vi "_SendTelemetry.vi"(5 "Bytes":u8, 6 "Output":refnum<k21>, 7 "Telemetry Offset":i16, 8 "error in (no error)":errorcluster, 9 "IP in":i16, 10 "Instructions":refnum<k21>, 11 "Telemetry FIFO":refnum<k21>) -> (0 "error out":errorcluster, 3 "IP out":i16)   [LabVIEW 2018, in "Modbus_Processing_Unit.lvlib" / "MPU.lvclass"]
uses:
  MPU.lvclass
  ts_m1m3supportFPGA/src/Common_FPGA_HealthAndStatus/DataTypes/HealthAndStatusUpdate.ctl
  ts_m1m3supportFPGA/src/Common_FPGA_HealthAndStatus/DataTypes/HealthAndStatusUpdateMode.ctl
  <vilib>/rvi/DataTransferAndStorage/Container/Common/niFpgaContainerExecOnDevCompGetState.vi
  <vilib>/rvi/Emulation/niFpgaEmulationIsFPGAContextNoSignature.vi
  <vilib>/rvi/DataTransferAndStorage/Container/Common/niFpgaContainerGetUniqueNameForEmu.vi
  <vilib>/rvi/Emulation/niFpgaProcessEmulError.vi
  <vilib>/rvi/Emulation/niFpgaSctlEmulationGetInTimedLoop.vi
  <vilib>/rvi/errors/nirviReportUnexpectedCaseInternalError (U32).vi
  <vilib>/rvi/Memory/Memory_Emulation/niFpgaMemoryEmulationCacheClearOnFirstRun.vi
  <vilib>/rvi/Memory/Memory_Emulation/nirvimemoryEmulationManagerCache_MakeExclusive.vi
  <vilib>/rvi/Memory/Memory_Emulation/niFpgaMemoryEmulationValidateCache.vi
  <vilib>/rvi/Memory/Memory_Emulation/nirvimemoryEmulationManagerCache_InsertValue.vi
  <vilib>/Utility/error.llb/Clear Errors.vi
  <vilib>/rvi/Memory/Memory_Emulation/nirvimemoryEmulationManagerCache_ReleaseExclusive.vi
  <vilib>/rvi/Memory/Memory_Emulation/nirvimemoryEmulationManagerCache_GetValue.vi
  <vilib>/rvi/Memory/Memory_Emulation/nirvimemoryEmulationManagerCache_SetValue.vi
  <vilib>/rvi/Emulation/niFpgaSctlEmulationResourceMgr.vi
  <vilib>/rvi/errors/niFpgaSetErrorForExecOnDevCompSimple.vi
  <vilib>/rvi/eio/common/nirviEmuReportErrorAndStop.vi
  <vilib>/rvi/FIFO/Fifo_Resource/nirvififoEmulationSetSize.vi
  <vilib>/rvi/FIFO/Fifo_Resource/nirviFifoEmulationQueueMgr.vi
  <instcachedir>/0/nirviFifoEmulationQueueMgr_E5CAEC123FF24DC58D834DCA3CDAA9B5.lvgen/nirviFifoEmulationQueueMgr_E5CAEC123FF24DC58D834DCA3CDAA9B5_022.vi
  <vilib>/rvi/FIFO/Fifo_Resource/nirvififoEmulationDetermineInputValidOut.vi
  <vilib>/rvi/FIFO/Fifo_Resource/nirvififoEmulationCreateLock.vi
  <vilib>/rvi/FIFO/Fifo_Resource/nirvififoEmulationObtainLock.vi
  <vilib>/rvi/FIFO/Fifo_Resource/nirvififoEmulationReleaseLock.vi
  <vilib>/rvi/occurrence/nirviWaitOnOccurrenceBase.vi
  <vilib>/rvi/errors/nirviReportUnexpectedCaseInternalError.vi
  <vilib>/rvi/interface/RandomDataEmulation/niFpgaRandomDataHandleErrors.vi
  <vilib>/rvi/DataTransferAndStorage/Container/XNode/niFpgaContainer.xnode
  <vilib>/rvi/Memory/Memory_Emulation/niFpgaMemoryEmulationRefIn.vi
  <vilib>/rvi/FIFO/Fifo_Resource/niFpgaFifoEmulationRefIn.vi
  ts_m1m3supportFPGA/src/Common_FPGA_HealthAndStatus/FPGAHealthAndStatus.lvlib
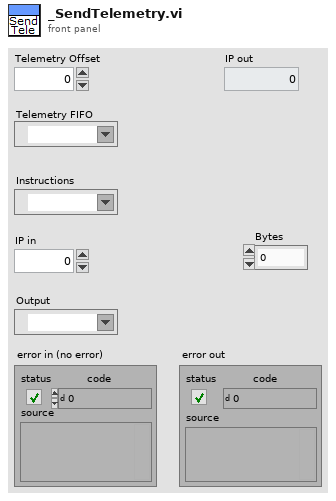
[diagram p1: front panel]
types:
  T1 = typedef "FPGAHealthAndStatus.lvlib/HealthAndStatusUpdate.ctl" = cluster{"Address":u32, "UpdateMode":T2, "Data":u64}
  T2 = typedef "FPGAHealthAndStatus.lvlib/HealthAndStatusUpdateMode.ctl" = enum8{"NOP", "Set", "Add", "Subtract", "Or", "Not And"}
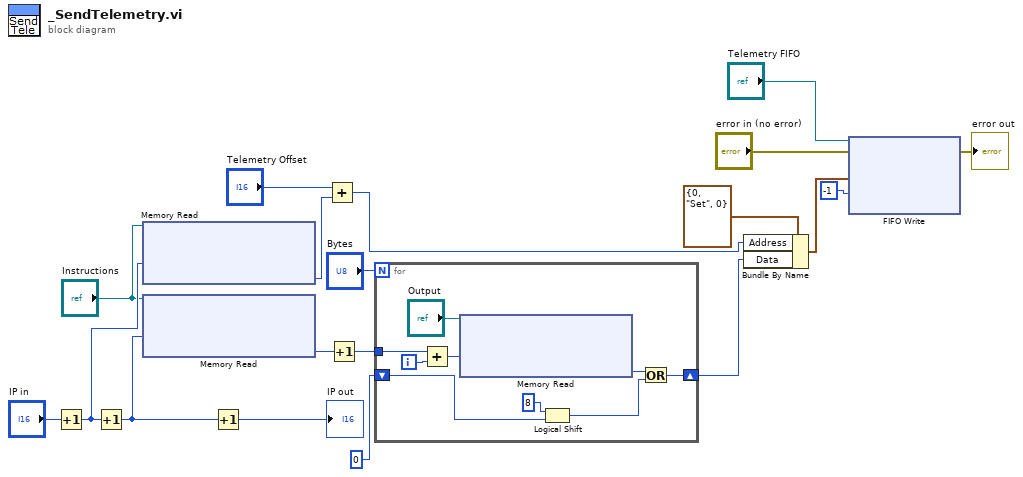
[diagram p0: block diagram]
diagram:
  n1 = Increment(x="IP in") -> (x+1=w5:i16)
  n2 = Increment(x=w5) -> (x+1=w2:i16)
  n3 = xnode ("Memory Read")("Address"=w5, "Memory In"="Instructions") -> ("Data"=w4:u8)  [unwired: 1 out]
  n4 = xnode ("Memory Read")("Address"=w2, "Memory In"="Instructions") -> ("Data"=w1:u8)  [unwired: 1 out]
  n5 = Increment(x=w2) -> (x+1=→"IP out":i16)
  n6 = Add(x="Telemetry Offset", y=w4) -> (x+y=w15:i16)
  n7 = Increment(x=w1) -> (x+1=w19:u8)
  n8 = for {
    N: "Bytes" -> [_]
    tunnel: w19 -> [w27]
    shift-right: [w23] -> w8
    shift-left: u64 0 -> [w26]
    i -> [w28]
    n9 = Add(x=w27, y=w28) -> (x+y=w21:i32)
    n10 = xnode ("Memory Read")("Address"=w21, "Memory In"="Output") -> ("Data"=w20:u8)  [unwired: 1 out]
    n11 = Logical Shift(y=i16 8, x=w26) -> (x << y=w24:u64)
    n12 = Or(x=w20, y=w24) -> (x .or. y?=w23:u64)
  }
  n13 = Bundle By Name(cluster=T1 {"Address"=0, "UpdateMode"=enum."Set", "Data"=0} ("HealthAndStatusUpdate"), "Address"=w15, "Data"=w8) -> (w13:T1)
  n14 = xnode ("FIFO Write")("Element"=w13, "Timeout"=-1, "error in (no error)"="error in (no error)", "FIFO In"="Telemetry FIFO") -> ("error out"=→"error out":errorcluster)  [unwired: 2 out]
